vi "MacroExecution.vi"(7 "MacroExecution Command":enum16{"Initialize", "Run"}(ring), 8 "Error In":errorcluster, 11 "Macro IN":string[](array[string])) -> (0 "Error Out":errorcluster, 1 "Skip?":bool, 2 "Paused?":bool, 3 "Execution Complete?":bool, 4 "Pause Duration":dbl, 5 "Current Execution Index":i32)   [LabVIEW 2012]
uses:
  Custom Controls and Typedefs/LOOP Control Cluster.ctl
panel:
  in  "Array 3":string[](array[string])=["LOOP.Start(iterations,2)", "Pause(wait.seconds,1)", "LOOP.Start(iterations,3)", "Pause(wait.seconds,2)", "LOOP.End", "LOOP.End", ""]
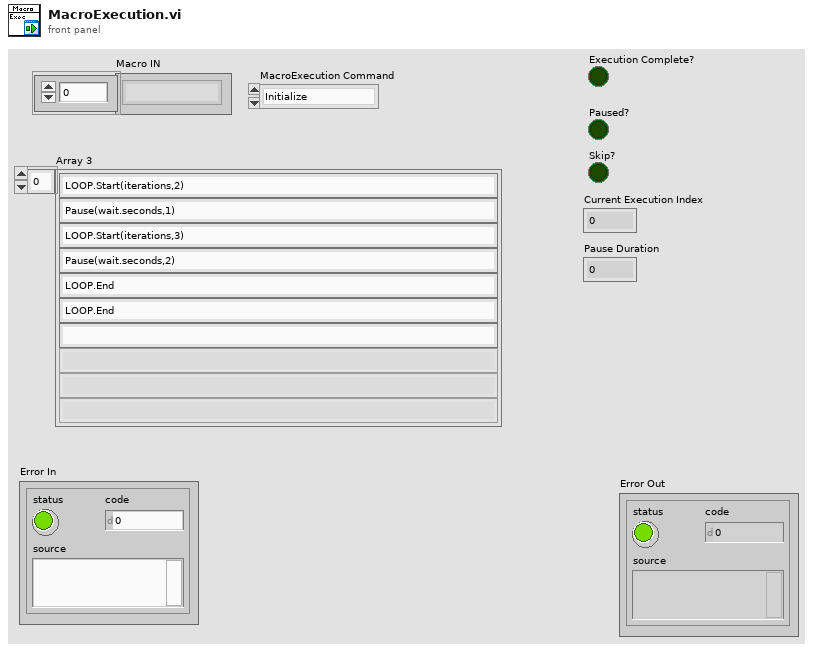
[diagram p1: front panel]
types:
  T1 = typedef "LOOP Control Cluster.ctl" = cluster{"Index of LOOP.Start":i32, "Iteration Count Down":i32}
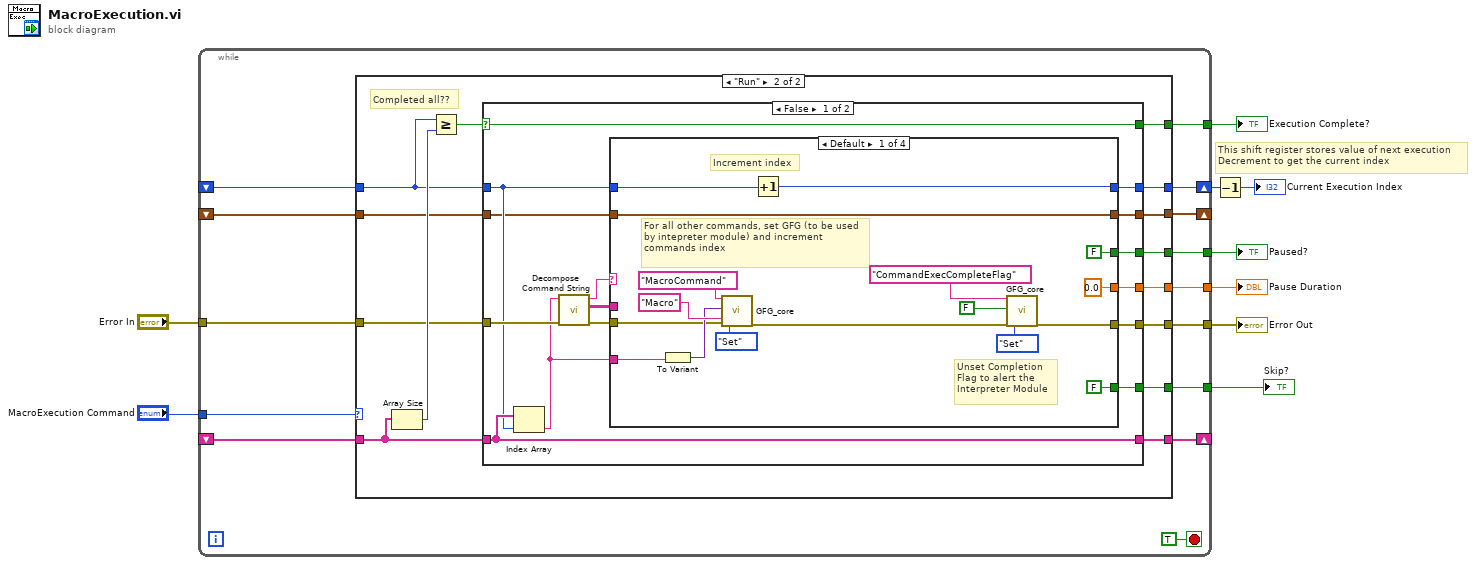
[diagram p0: block diagram]
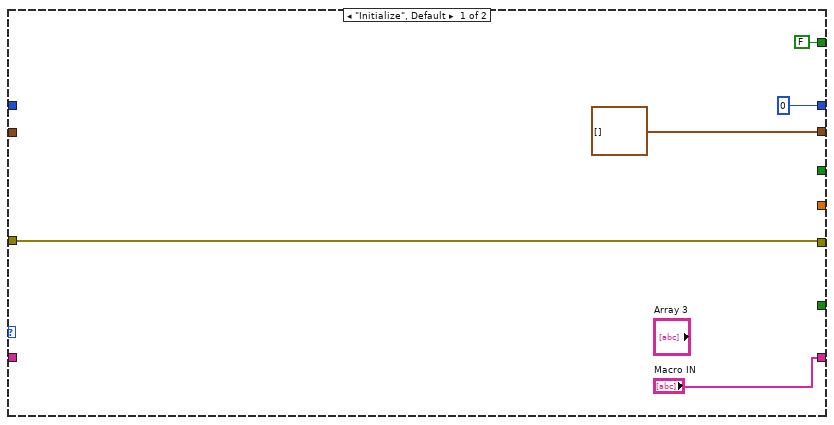
[diagram p2: hidden frame]
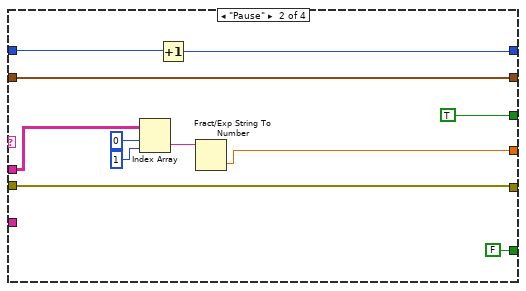
[diagram p3: hidden frame]
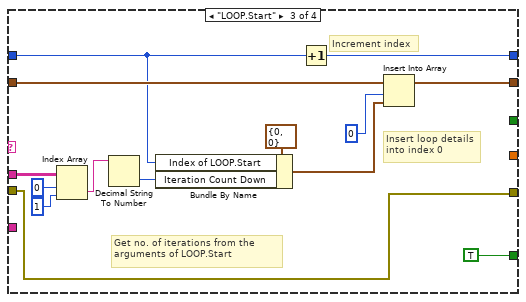
[diagram p4: hidden frame]
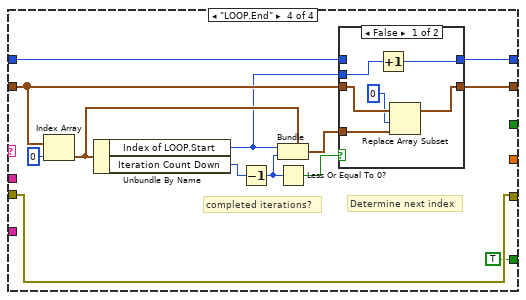
[diagram p5: hidden frame]
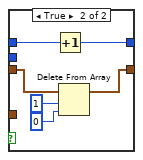
[diagram p6: hidden frame]
diagram:
  # "This shift register stores value of next execution\nDecrement to get the current index"
  n1 = while {
    shift-right: [w18] -> w2
    shift-left: _ -> [w23]
    tunnel: [w20] -> w9
    tunnel: "MacroExecution Command" -> [w19]
    shift-right: [w17] -> _
    shift-left: _ -> [w22]
    shift-right: [w15] -> _
    shift-left: _ -> [w16]
    tunnel: "Error In" -> [w14]
    tunnel: [w13] -> w6
    tunnel: [w12] -> w5
    tunnel: [w11] -> w4
    tunnel: [w10] -> w3
    stop <- TRUE stop-if-true
    n2 = case shown="\"Run\"" w19 {
      tunnel: w23 -> [_ w41]
      tunnel: w22 -> [_ w40]
      tunnel: [FALSE w38] -> w20
      tunnel: [0 w33] -> w18
      tunnel: ["Macro IN" w37] -> w17
      tunnel: w16 -> [_ w36]
      tunnel: [T1[] [] w34] -> w15
      tunnel: w14 -> [w25 w35]
      tunnel: [w25 w32] -> w13
      tunnel: [_ w31] -> w12
      tunnel: [_ w30] -> w11
      tunnel: [_ w29] -> w10
      frame "Initialize", Default {
      }
      frame "Run" {
        # "Completed all??"
        n3 = Array Size(array=w40) -> (size(s)=w42:i32)
        n4 = Greater Or Equal?(x=w41, y=w42) -> (x >= y?=w39:bool)
        n5 = case shown="False" w39 {
          selector: w39 -> [w57 w128]
          tunnel: w41 -> [w52 w125]
          tunnel: w40 -> [w56 w129]
          tunnel: [w57 w128] -> w38
          tunnel: [w56 w129] -> w37
          tunnel: w36 -> [w51 w126]
          tunnel: w35 -> [w55 w127]
          tunnel: [w50 w126] -> w34
          tunnel: [w49 w125] -> w33
          tunnel: [w48 w127] -> w32
          tunnel: [w45 _] -> w31
          tunnel: [w44 _] -> w30
          tunnel: [w43 _] -> w29
          frame False {
            n6 = Index Array(array=w56, index=w52) -> (element=w47:string)
            n7 = call "Decompose Command String.vi"("Error In"=w55, "Command IN"=w47) -> ("Error Out"=w53:errorcluster, "ArgumentTable"=w46:string[][], "Action"=w54:string)  [unwired: 7 in]
            n8 = case shown="Default" w54 {
              tunnel: w53 -> [w65 w76 w88 w107]
              tunnel: w52 -> [w74 w84 w90 w103]
              tunnel: w51 -> [w72 w85 w94 w109]
              tunnel: [w72 w85 w92 w108] -> w50
              tunnel: [w73 w83 w89 w102] -> w49
              tunnel: [w61 w76 w88 w107] -> w48
              tunnel: w47 -> [w68 _ _ _]
              tunnel: w46 -> [_ w81 w87 _]
              tunnel: [FALSE TRUE _ _] -> w45
              tunnel: [0.0 w77 _ _] -> w44
              tunnel: [FALSE ("Skip?") FALSE ("Skip?") TRUE ("Skip?") TRUE ("Skip?")] -> w43
              frame Default {
                # "Unset Completion Flag to alert the Interpreter Module"
                # "For all other commands, set GFG (to be used by intepreter module) and increment commands index"
                # "Increment index"
                n9 = To Variant(anything=w68) -> (Variant=w69:variant)
                n10 = call "GFG_core.vi"("Variable Name in"="MacroCommand" ("Source VI"), "Variant in"=w69, "Source VI"="Macro", "error in (no error)"=w65, "Action"=enum16{"Init", "Set", "Get", "Clear"}."Set") -> ("error out"=w60:errorcluster)  [unwired: 8 in, 6 out]
                n11 = Increment(x=w74) -> (x+1=w73:i32)
                n12 = call "GFG_core.vi"("Variable Name in"="CommandExecCompleteFlag", "Variant in"=FALSE, "error in (no error)"=w60, "Action"=enum16{"Init", "Set", "Get", "Clear"}."Set") -> ("error out"=w61:errorcluster)  [unwired: 9 in, 6 out]
              }
              frame "Pause" {
                n13 = Index Array(array=w81, index (row)=0, index (col)=1 ("disabled index (col)")) -> (element=w78:string)
                n14 = Increment(x=w84) -> (x+1=w83:i32)
                n15 = Fract/Exp String To Number(string=w78) -> (number=w77:dbl)  [unwired: 3 in, 1 out]
              }
              frame "LOOP.Start" {
                # "Increment index"
                # "Insert loop details into index 0"
                # "Get no. of iterations from the arguments of LOOP.Start"
                n16 = Index Array(array=w87, index (row)=0, index (col)=1 ("disabled index (col)")) -> (element=w96:string)
                n17 = Decimal String To Number(string=w96) -> (number=w95:i32)  [unwired: 2 in, 1 out]
                n18 = Bundle By Name(cluster=T1 {"Index of LOOP.Start"=0, "Iteration Count Down"=0} ("LOOP Control Cluster"), "Index of LOOP.Start"=w90, "Iteration Count Down"=w95) -> (w93:T1)
                n19 = Increment(x=w90) -> (x+1=w89:i32)
                n20 = Insert Into Array(array=w94, index=0, new element=w93) -> (w92:T1[])
              }
              frame "LOOP.End" {
                # "Determine next index"
                # "completed iterations?"
                n21 = Index Array(array=w109, index=0) -> (element=w106:T1)
                n22 = Unbundle By Name(w106) -> ("Index of LOOP.Start"=w101:i32, "Iteration Count Down"=w111:i32)
                n23 = Decrement(x=w111) -> (x-1=w105:i32)
                n24 = Bundle(cluster=w106, "Index of LOOP.Start"=w101, "Iteration Count Down"=w105) -> (w104:T1)
                n25 = Less Or Equal To 0?(x=w105) -> (x <= 0?=w110:bool)
                n26 = case shown="False" w110 {
                  tunnel: w109 -> [w118 w124]
                  tunnel: [w115 w123] -> w108
                  tunnel: w104 -> [w116 _]
                  tunnel: w103 -> [_ w120]
                  tunnel: [w113 w119] -> w102
                  tunnel: w101 -> [w114 _]
                  frame False {
                    n27 = Increment(x=w114) -> (x+1=w113:i32)
                    n28 = Replace Array Subset(array=w118, new element=w116, index=0) -> (w115:T1[])
                  }
                  frame True {
                    n29 = Increment(x=w120) -> (x+1=w119:i32)
                    n30 = Delete From Array(array=w124, length=1, index=0) -> (array with subset deleted=w123:T1[])  [unwired: 1 out]
                  }
                }
              }
            }
          }
          frame True {
          }
        }
      }
    }
  }
  "Error Out" <- w6
  "Execution Complete?" <- w9
  "Paused?" <- w5
  "Pause Duration" <- w4
  "Skip?" <- w3
  n31 = Decrement(x=w2) -> (x-1=→"Current Execution Index":i32)
